vi "vaa3d call.vi"() -> ()   [LabVIEW 2020]
panel:
  in  "Call_Vaa3D 2":bool
  in  "spacing_between_points":dbl=10.0 min=0.05 max=100.0 step=1.0 format="%#.3f"
  in  "Call_Vaa3D":bool caption="Load\nolder\nPOI"
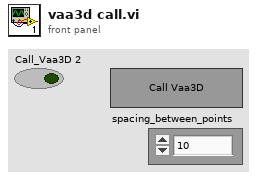
[diagram p1: front panel]
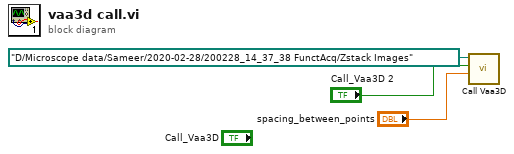
[diagram p0: block diagram]
diagram:
  n1 = call "Call Vaa3D.vi"("spacing_between_points"="spacing_between_points", "Call_Vaa3D"="Call_Vaa3D 2", "Z-stack folder path"=path "D:/Microscope data/Sameer/2020-02-28/200228_14_37_38 FunctAcq/Zstack Images") -> ()  [unwired: 8 in, 1 out]
